vi "队列次vi.vi"() -> ()   [LabVIEW 2024]
uses:
  <vilib>/sound2/lvsound2.llb/Sound Data Format.ctl
  <vilib>/sound2/lvsound2.llb/Sampling Mode.ctl
  <vilib>/sound2/lvsound2.llb/Sound File Info (path).vi
  <vilib>/sound2/lvsound2.llb/Sound File Read Open.vi
  <vilib>/sound2/lvsound2.llb/Sound File Read (DBL).vi
  <vilib>/sound2/lvsound2.llb/Sound Output Write (DBL).vi
  <vilib>/sound2/lvsound2.llb/Sound File Write Open.vi
  <vilib>/sound2/lvsound2.llb/Sound Input Read (DBL).vi
  <vilib>/express/express analysis/Spectral/Block/exnSpectralBlock spectral measurements RMS poly.vi
  <vilib>/express/express analysis/Spectral/Block/exnSpectralBlock spectral measurements RMS array WFM.vi
  <vilib>/sound2/lvsound2.llb/Sound File Write (DBL).vi
  <vilib>/express/express analysis/Spectral/XNode/ExpressSpectralMeasurementsBlockNode.xnode
panel:
  out "布尔 2":bool
  out "布尔":bool
  in  "device ID 3":u32 caption="设备ID"
  in  "number of samples/ch 3":i32=100000 caption="每通道采样数"
  in  "number of samples/ch":i32=100000 caption="每通道采样数"
  in  "sample mode":T1=1 caption="采样模式" items=["有限采样", "连续采样"]
  in  "sound format":T2={"sample rate (S/s)"=22050.0, "number of channels"=2, "bits per sample"=16} caption="声音格式"
  in  "device ID":u32 caption="设备ID"
  out "error out":errorcluster caption="错误输出"
  in  "?":enum32{"选项卡 1", "选项卡 2"}(tab)
  out "波形图":waveform(dbl)[](graph)
  out "波形图 2":cluster{"f0":dbl, "df":dbl, "magnitude":dbl[]}[](graph)
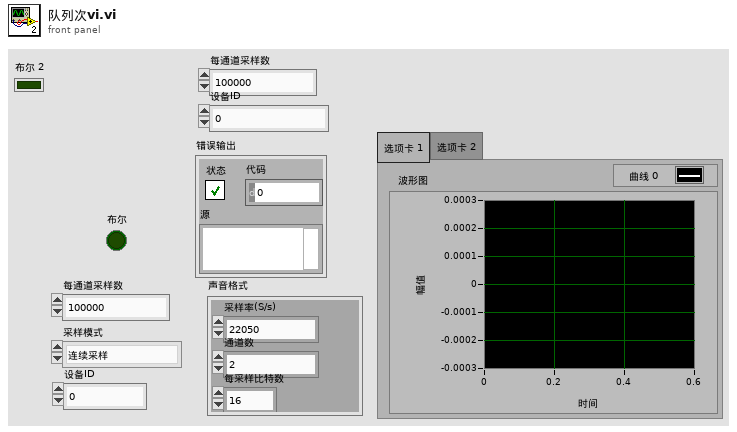
[diagram p1: front panel]
types:
  T1 = typedef "Sampling Mode.ctl" = i32
  T2 = typedef "Sound Data Format.ctl" = cluster{"sample rate (S/s)":dbl, "number of channels":i32, "bits per sample":i32}
  T3 = typedef "Sound Output Task ID.ctl" = u32
  T4 = typedef "Sound File Refnum.ctl" = refnum<file>
  T5 = cluster{"averaging mode":u16, "weighting mode":u16, "number of averages":u32}
  T6 = cluster{"dB On (F)":bool, "unwrap phase (F)":bool, "convert to degree (F)":bool}
  T7 = typedef "Sound Input Task ID.ctl" = u32
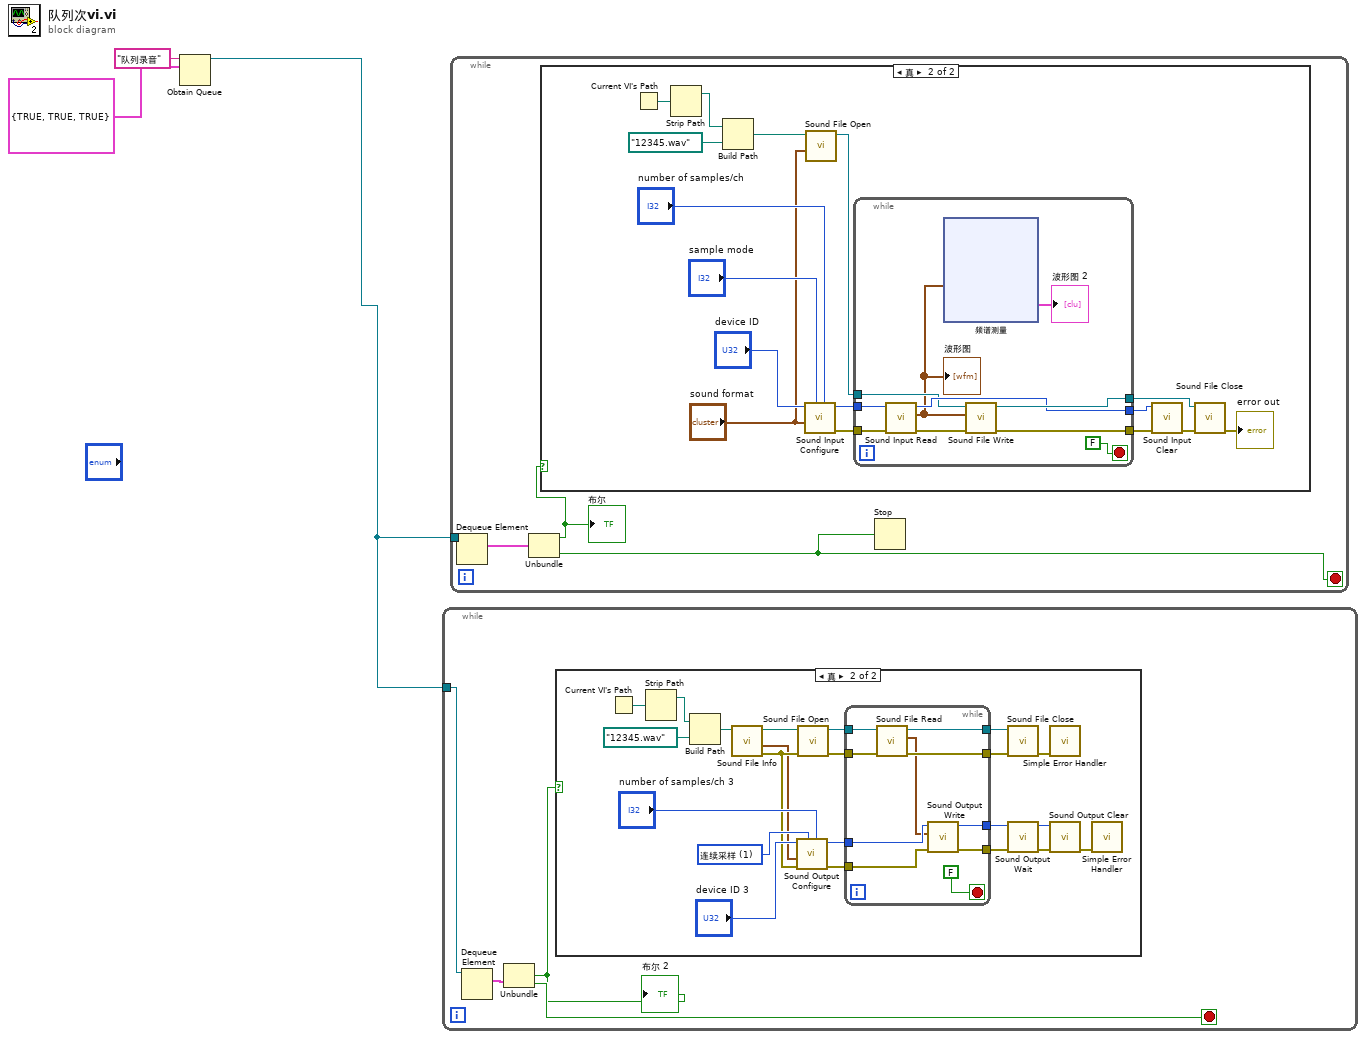
[diagram p0: block diagram]
diagram:
  n1 = Obtain Queue(name (unnamed)="队列录音" ("名称（未命名）"), element data type=cluster{bool, bool, bool} {TRUE, TRUE, TRUE}) -> (queue out=w1:refnum<queue>)  [unwired: 3 in, 2 out]
  n2 = while {
    tunnel: w1 -> [w7]
    stop <- w5 stop-if-true
    n3 = Dequeue Element(queue=w7) -> (element=w6:cluster{bool, bool, bool})  [unwired: 2 in, 3 out]
    n4 = Unbundle(w6) -> (w4:bool, w5:bool)  [unwired: 1 out]
    "布尔 2" <- w4
    n5 = case shown="真" w4 {
      frame False {
      }
      frame True {
        w18 = T1 1 items=["有限采样", "连续采样"] ("sample mode")
        n6 = Current VI's Path() -> (path=w29:path)
        n7 = Strip Path(path=w29) -> (stripped path=w28:path)  [unwired: 1 out]
        n8 = Build Path(base path=w28, name or relative path=path "12345.wav" ("名称或相对路径")) -> (appended path=w26:path)
        n9 = call-poly <vilib>:"Sound File Info.vi"("path"=w26) -> ("error out"=w17:errorcluster, "sound format"=w8:T2, "path out"=w23:path)  [unwired: 7 in, 1 out]
        n10 = call <vilib>:"Sound Output Configure.vi"("number of samples/ch"="number of samples/ch 3", "sample mode"=w18, "error in (no error)"=w17, "sound format"=w8, "device ID"="device ID 3") -> ("error out"=w16:errorcluster, "task ID"=w11:T3)  [unwired: 5 in]
        n11 = call-poly <vilib>:"Sound File Open.vi"("error in (no error)"=w17, "path"=w23) -> ("error out"=w25:errorcluster, "sound file refnum"=w22:T4)  [unwired: 8 in]
        n12 = while {
          tunnel: w25 -> [w39]
          tunnel: [w38] -> w24
          tunnel: w22 -> [w37]
          tunnel: [w36] -> w21
          tunnel: w16 -> [w35]
          tunnel: [w34] -> w15
          tunnel: w11 -> [w32]
          tunnel: [w31] -> w10
          stop <- FALSE stop-if-true
          n13 = call-poly <vilib>:"Sound File Read.vi"("error in (no error)"=w39, "sound file refnum"=w37) -> ("error out"=w38:errorcluster, "data"=w30:waveform(dbl)[], "sound file refnum out"=w36:T4)  [unwired: 5 in, 2 out]
          n14 = call-poly <vilib>:"Sound Output Write.vi"("error in (no error)"=w35, "data"=w30, "task ID"=w32) -> ("error out"=w34:errorcluster, "task ID out"=w31:T3)  [unwired: 7 in]
        }
        n15 = call <vilib>:"Sound File Close.vi"("error in (no error)"=w24, "sound file refnum"=w21) -> ("error out"=w13:errorcluster)  [unwired: 9 in]
        n16 = call <vilib>:"Sound Output Wait.vi"("error in (no error)"=w15, "task ID"=w10) -> ("error out"=w14:errorcluster, "task ID out"=w9:T3)  [unwired: 8 in]
        n17 = call <vilib>:"Simple Error Handler.vi"("error in (no error)"=w13) -> ()  [unwired: 4 in, 5 out]
        n18 = call <vilib>:"Sound Output Clear.vi"("error in (no error)"=w14, "task ID"=w9) -> ("error out"=w12:errorcluster)  [unwired: 9 in]
        n19 = call <vilib>:"Simple Error Handler.vi"("error in (no error)"=w12) -> ()  [unwired: 4 in, 5 out]
      }
    }
  }
  n20 = while {
    tunnel: w1 -> [w43]
    stop <- w40 stop-if-true
    n21 = Dequeue Element(queue=w43) -> (element=w42:cluster{bool, bool, bool})  [unwired: 2 in, 3 out]
    n22 = Unbundle(w42) -> (w41:bool, w40:bool)  [unwired: 1 out]
    "布尔" <- w41
    n23 = case shown="真" w41 {
      frame False {
      }
      frame True {
        n24 = Current VI's Path() -> (path=w50:path)
        n25 = Strip Path(path=w50) -> (stripped path=w49:path)  [unwired: 1 out]
        n26 = Build Path(base path=w49, name or relative path=path "12345.wav" ("名称或相对路径")) -> (appended path=w48:path)
        n27 = call <vilib>:"Sound Input Configure.vi"("number of samples/ch"="number of samples/ch", "sample mode"="sample mode", "sound format"="sound format", "device ID"="device ID") -> ("error out"=w56:errorcluster, "task ID"=w52:T7)  [unwired: 6 in]
        n28 = call-poly <vilib>:"Sound File Open.vi"("sound format"="sound format", "path"=w48) -> ("sound file refnum"=w47:T4)  [unwired: 8 in, 1 out]
        n29 = while {
          tunnel: [w66] -> w53
          tunnel: w47 -> [w63]
          tunnel: w56 -> [w69]
          tunnel: [w67] -> w55
          tunnel: w52 -> [w65]
          tunnel: [w64] -> w51
          stop <- FALSE stop-if-true
          n30 = call-poly <vilib>:"Sound Input Read.vi"("error in (no error)"=w69, "task ID"=w65) -> ("error out"=w68:errorcluster, "data"=w62:waveform(dbl)[], "task ID out"=w64:T7)  [unwired: 7 in]
          "波形图" <- w62
          n31 = xnode "频谱测量"("信号"=w62) -> ("测量输出"=→"波形图 2":cluster{"f0":dbl, "df":dbl, "magnitude":dbl[]}[])  [unwired: 1 in, 2 out]
          n32 = call-poly <vilib>:"Sound File Write.vi"("error in (no error)"=w68, "data"=w62, "sound file refnum"=w63) -> ("error out"=w67:errorcluster, "sound file refnum out"=w66:T4)  [unwired: 7 in]
        }
        n33 = call <vilib>:"Sound Input Clear.vi"("error in (no error)"=w55, "task ID"=w51) -> ("error out"=w54:errorcluster)  [unwired: 9 in]
        n34 = call <vilib>:"Sound File Close.vi"("error in (no error)"=w54, "sound file refnum"=w53) -> ("error out"=→"error out":errorcluster)  [unwired: 9 in]
      }
    }
    n35 = Stop(stop? (T)=w40) -> ()
  }
